vi "VelocityControl.vi"(0 "estimatives":T3, 1 "Dest_orientation":dbl, 2 "Position":dbl[](array[numeric]), 3 "Waypoint 1":dbl[](array[numeric]), 4 "Waypoint 0":dbl[](array[numeric]), 5 "Vx":dbl format="%#_13g", 9 "Vy":dbl format="%#_13g", 11 "output xy":dbl=2.4, 12 "output inc":dbl=2.4, 13 "output angle":dbl=4.0) -> (8 "Output Velocity":dbl[](array[numeric]) format="%.2f")   [LabVIEW 2017]
uses:
  Controle/VelocityGraph.ctl
  <vilib>/Analysis/coordinate.llb/Wrap Angle (scalar).vi
  <vilib>/Analysis/coordinate.llb/2D Cartesian Coordinate Rotation (Scalar).vi
  <vilib>/Analysis/NI_AAL_Angle.lvlib
  <vilib>/Analysis/NI_AALPro.lvlib
panel:
  out "Velocity Y":T1
  out "Velocity X":T1
  in  "PID gains Vel":T2={"proportional gain (Kc)"=0.3, "integral time (Ti, min)"=0.0, "derivative time (Td, min)"=0.001}
  in  "PID Gains Angle":T2={"proportional gain (Kc)"=5.0, "integral time (Ti, min)"=0.0, "derivative time (Td, min)"=-2.0}
  in  "Reinitialize":bool
  in  "PID Gains lateral":T2={"proportional gain (Kc)"=8e-05, "integral time (Ti, min)"=0.0, "derivative time (Td, min)"=-0.07}
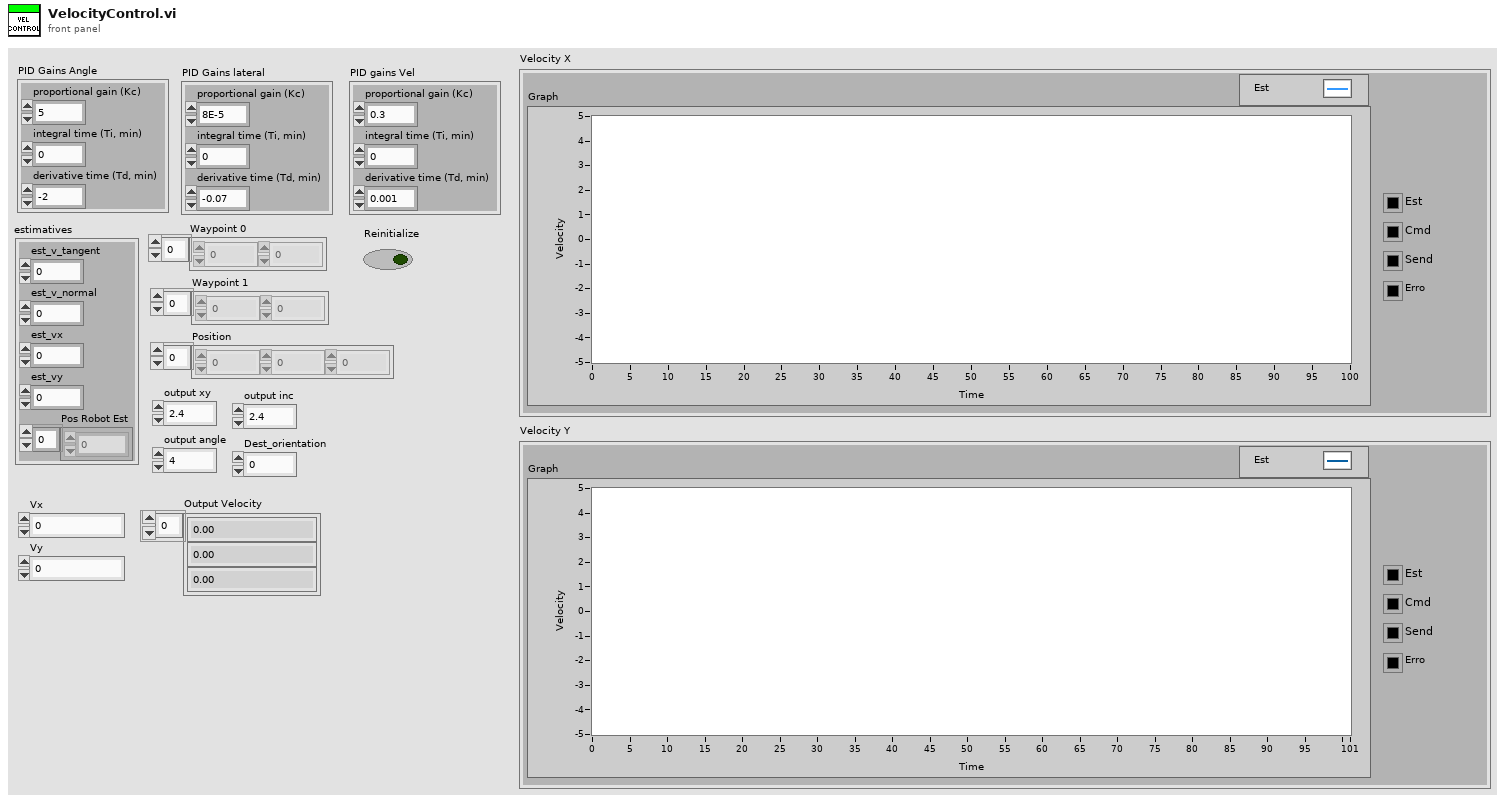
[diagram p1: front panel]
types:
  T1 = typedef "VelocityGraph.ctl" = cluster{"Graph":cluster{"est_vx":dbl, "Vx":dbl, dbl, "x out":dbl}, "Est":u32, "Cmd":u32, "Send":u32, "Erro":u32}
  T2 = cluster{"proportional gain (Kc)":dbl, "integral time (Ti, min)":dbl, "derivative time (Td, min)":dbl}
  T3 = cluster{"est_v_tangent":dbl, "est_v_normal":dbl, "est_vx":dbl, "est_vy":dbl, "Pos Robot Est":dbl[]}
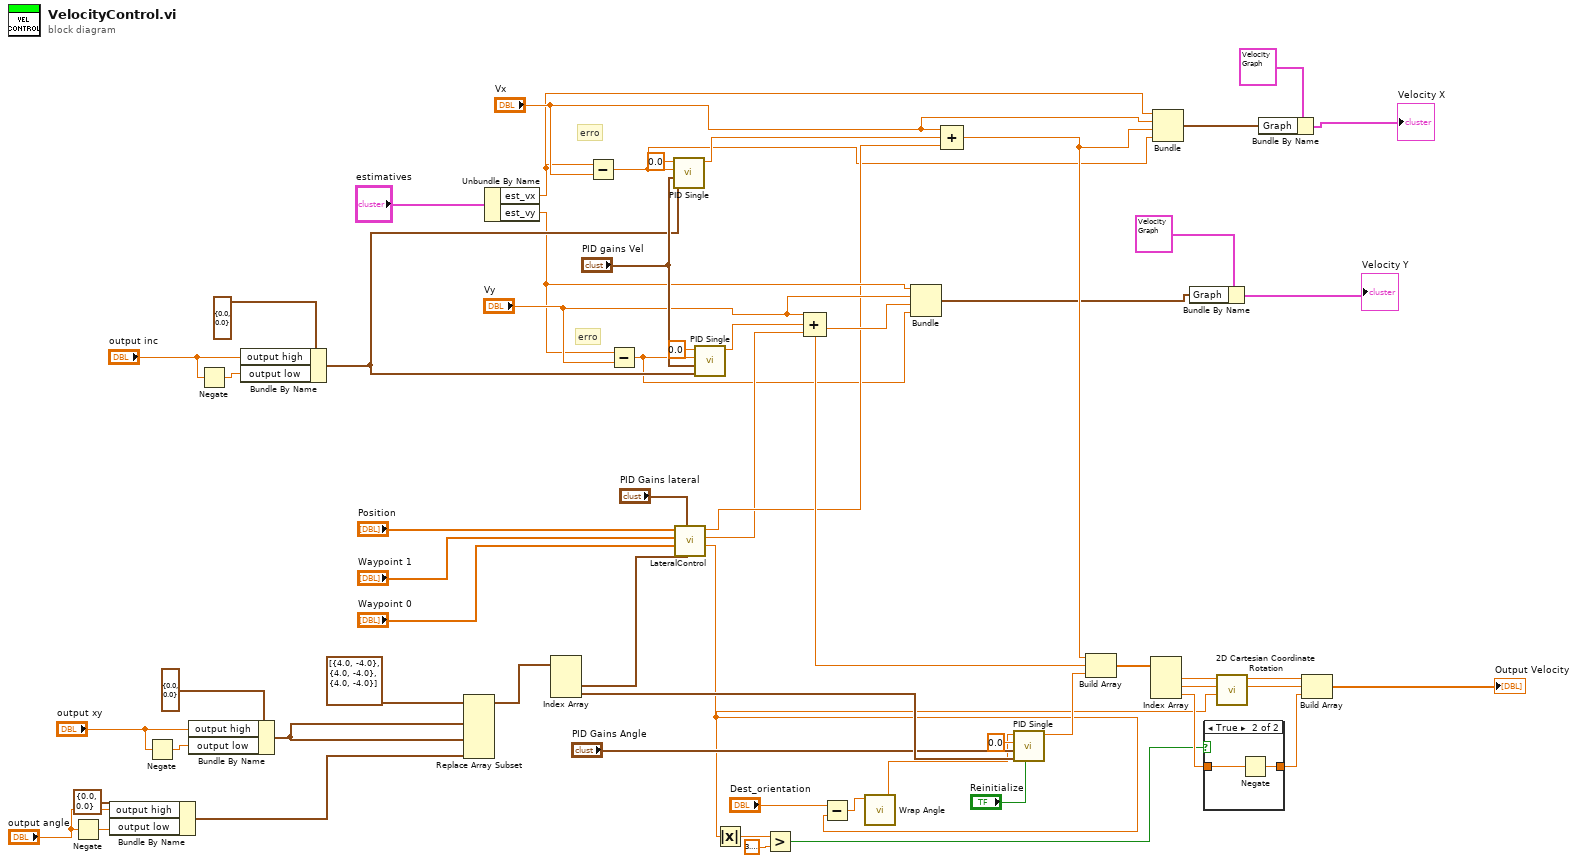
[diagram p0: block diagram]
diagram:
  # "erro"
  # "erro"
  n1 = Negate(x="output angle") -> (-x=w37:dbl)
  n2 = Bundle By Name(cluster=cluster{"output high":dbl, "output low":dbl} {"output high"=0.0, "output low"=0.0}, "output high"="output angle", "output low"=w37) -> (w43:cluster{"output high":dbl, "output low":dbl})
  n3 = Negate(x="output xy") -> (-x=w39:dbl)
  n4 = Bundle By Name(cluster=cluster{"output high":dbl, "output low":dbl} {"output high"=0.0, "output low"=0.0} ("new element/subarray"), "output high"="output xy", "output low"=w39) -> (w41:cluster{"output high":dbl, "output low":dbl})
  n5 = Negate(x="output inc") -> (-x=w15:dbl)
  n6 = Bundle By Name(cluster=cluster{"output high":dbl, "output low":dbl} {"output high"=0.0, "output low"=0.0} ("new element/subarray"), "output high"="output inc", "output low"=w15) -> (w13:cluster{"output high":dbl, "output low":dbl})
  n7 = Replace Array Subset(array=cluster{"output high":dbl, "output low":dbl}[] [{"output high"=4.0, "output low"=-4.0}, {"output high"=4.0, "output low"=-4.0}, {"output high"=4.0, "output low"=-4.0}] ("output range"), new element #1=w41, new element #2=w41, new element #3=w43) -> (w40:cluster{"output high":dbl, "output low":dbl}[])  [unwired: 3 in]
  n8 = Unbundle By Name("estimatives") -> ("est_vx"=w12:dbl, "est_vy"=w11:dbl)
  n9 = Index Array(array=w40) -> (element #2=w27:cluster{"output high":dbl, "output low":dbl}, element #3=w51:cluster{"output high":dbl, "output low":dbl})  [unwired: 3 in, 1 out]
  n10 = Subtract(x=w12, y="Vx") -> (x-y=w2:dbl)
  n11 = Subtract(x=w11, y="Vy") -> (x-y=w1:dbl)
  n12 = call "PID Single.vi"("Limits"=w13, "PID gains in"="PID gains Vel", "Variable"=w2, "Setpoint"=0.0) -> ("Out"=w24:dbl)  [unwired: 7 in]
  n13 = call "LateralControl.vi"("output range"=w27, "PID Gains lateral"="PID Gains lateral", "Waypoint 0"="Waypoint 0", "Waypoint 1"="Waypoint 1", "Position"="Position") -> ("Numeric"=w34:dbl, "y out"=w9:dbl, "x out"=w10:dbl)  [unwired: 4 in]
  n14 = call "PID Single.vi"("Limits"=w13, "PID gains in"="PID gains Vel", "Variable"=w1, "Setpoint"=0.0) -> ("Out"=w23:dbl)  [unwired: 7 in]
  n15 = Absolute Value(x=w34) -> (abs(x)=w57:dbl)
  n16 = Greater?(x=w57, y=3.141592653589793) -> (0:w52:bool)
  n17 = Compound Arithmetic op=ADD("Vy", w23, w9) -> (w17:dbl)
  n18 = Subtract(x="Dest_orientation", y=w34) -> (x-y=w48:dbl)
  n19 = call-poly <vilib>:"Wrap Angle.vi"("angle in"=w48) -> ("angle out"=w47:dbl)  [unwired: 9 in, 1 out]
  n20 = Bundle("est_vy"=w11, "Vy"="Vy", w17, w1) -> (w7:cluster{"est_vy":dbl, "Vy":dbl, dbl, dbl})  [unwired: 1 in]
  n21 = Compound Arithmetic op=ADD("Vx", w24, w10) -> (w19:dbl)
  n22 = call "PID Single.vi"("initialize"="Reinitialize", "Limits"=w51, "PID gains in"="PID Gains Angle", "Variable"=0.0, "Setpoint"=w47) -> ("Out"=w53:dbl)  [unwired: 6 in]
  n23 = Build Array(w19, w17, w53) -> (w46:dbl[])
  n24 = Index Array(array=w46) -> (element #1=w61:dbl, element #2=w60:dbl, element #3=w56:dbl)  [unwired: 3 in]
  n25 = Bundle("est_vx"=w12, "Vx"="Vx", w19, w2) -> (w4:cluster{"est_vx":dbl, "Vx":dbl, dbl, dbl})  [unwired: 1 in]
  n26 = Bundle By Name(cluster=T1 {"Graph"={"est_vx"=-0.14571416207204627, "Vx"=0.4692407651588243, 1.5797768746041183, "x out"=1.110536109445294}, "Est"=16860, "Cmd"=16711680, "Send"=6618880, "Erro"=16776722} ("Velocity Y"), "Graph"=w7) -> (→"Velocity Y":T1)
  n27 = case shown="True" w52 {
    tunnel: w56 -> [w62 w64]
    tunnel: [w62 w63] -> w55
    frame False {
    }
    frame True {
      n28 = Negate(x=w64) -> (-x=w63:dbl)
    }
  }
  n29 = call-poly <vilib>:"2D Cartesian Coordinate Rotation.vi"("theta"=w34, "y"=w60, "x"=w61) -> ("y out"=w58:dbl, "x out"=w59:dbl)  [unwired: 6 in, 1 out]
  n30 = Bundle By Name(cluster=T1 {"Graph"={"est_vx"=-0.14571416207204627, "Vx"=0.4692407651588243, 1.5797768746041183, "x out"=1.110536109445294}, "Est"=16860, "Cmd"=16711680, "Send"=6618880, "Erro"=16776722} ("Velocity Y"), "Graph"=w4) -> (→"Velocity X":T1)
  n31 = Build Array(w59, w58, w55) -> (→"Output Velocity":dbl[])
